vi "SP Convert SP TDMS Graphics to Display Cluster.vi"(8 "error in (no error)":errorcluster, 9 "S Parameter Formatting":T9 {"Plots"."Ch 2"."Reference" format="%#.2g"; "Plots"."Ch 2"."Display Data" items=["Data", "Memory", "Data/Memory"]; "Plots"."Ch 2"."Format" items=["Log Mag", "Phase", "Expanded Phase", "Delay", "Smith", "Polar", "Lin Mag", "SWR", "Loss", "Real", "Imaginary"]; "Plots"."Ch 2"."Scale" min=0.001 step=1.0 format="%#.2g"; "Plots"."Ch 2"."Position" min=0.0 max=10.0; "Plots"."Ch 1"."Reference" format="%#.2g"; "Plots"."Ch 1"."Display Data" items=["Data", "Memory", "Data/Memory"]; "Plots"."Ch 1"."Format" items=["Log Mag", "Phase", "Expanded Phase", "Delay", "Smith", "Polar", "Lin Mag", "SWR", "Loss", "Real", "Imaginary"]; "Plots"."Ch 1"."Scale" min=0.001 step=1.0 format="%#.2g"; "Plots"."Ch 1"."Position" min=0.0 max=10.0}) -> (0 "error out":errorcluster, 3 "Display":T1={"Lock Control"=FALSE, "Retain Settings"=TRUE, "Formatted Data"=FALSE, "Plot Orientation"=enum."Single", "Plot Controls"=[{"Trace Orientation"=enum."Overlay", "Frequency"={"Change Frequency"=FALSE, "Start"=500.0, "Stop"=1500.0, "Units"=enum."MHz"}, "Markers"=[], "Traces"=[]}, {"Trace Orientation"=enum."Overlay", "Frequency"={"Change Frequency"=FALSE, "Start"=500.0, "Stop"=1500.0, "Units"=enum."MHz"}, "Markers"=[], "Traces"=[]}, {"Trace Orientation"=enum."Overlay", "Frequency"={"Change Frequency"=FALSE, "Start"=500.0, "Stop"=1500.0, "Units"=enum."MHz"}, "Markers"=[], "Traces"=[]}, {"Trace Orientation"=enum."Overlay", "Frequency"={"Change Frequency"=FALSE, "Start"=500.0, "Stop"=1500.0, "Units"=enum."MHz"}, "Markers"=[], "Traces"=[]}]} {"Plot Controls"."Traces"."Reference" format="%#.2g"; "Plot Controls"."Traces"."Display Data" items=["Data", "Memory", "Data/Memory"]; "Plot Controls"."Traces"."Format" items=["Log Mag", "Phase", "Expanded Phase", "Delay", "Smith", "Polar", "Lin Mag", "SWR", "Loss", "Real", "Imaginary"]; "Plot Controls"."Traces"."Scale" min=0.001 step=1.0 format="%#.2g"; "Plot Controls"."Traces"."Position" min=0.0 max=10.0; "Plot Controls"."Frequency"."Stop" format="%.3g"; "Plot Controls"."Frequency"."Start" format="%.3g"})   [LabVIEW 2011]
uses:
  TypeDefs/SP Formatting.ctl
  TypeDefs/SP Plot Orientation.ctl
  TypeDefs/SP Plot.ctl
  TypeDefs/SP Trace Orientation.ctl
  TypeDefs/SP Display Trace Controls.ctl
  TypeDefs/SP Display Format.ctl
  TypeDefs/SP Display Data.ctl
  TypeDefs/SP Frequency Units.ctl
  TypeDefs/SP Display Parameters.ctl
  TypeDefs/SP Display Plot Controls Cluster.ctl
  TypeDefs/SP Marker Cluster.ctl
  TypeDefs/SP Marker Type.ctl
panel:
  # "Div"
  # "Div"
  # "Div"
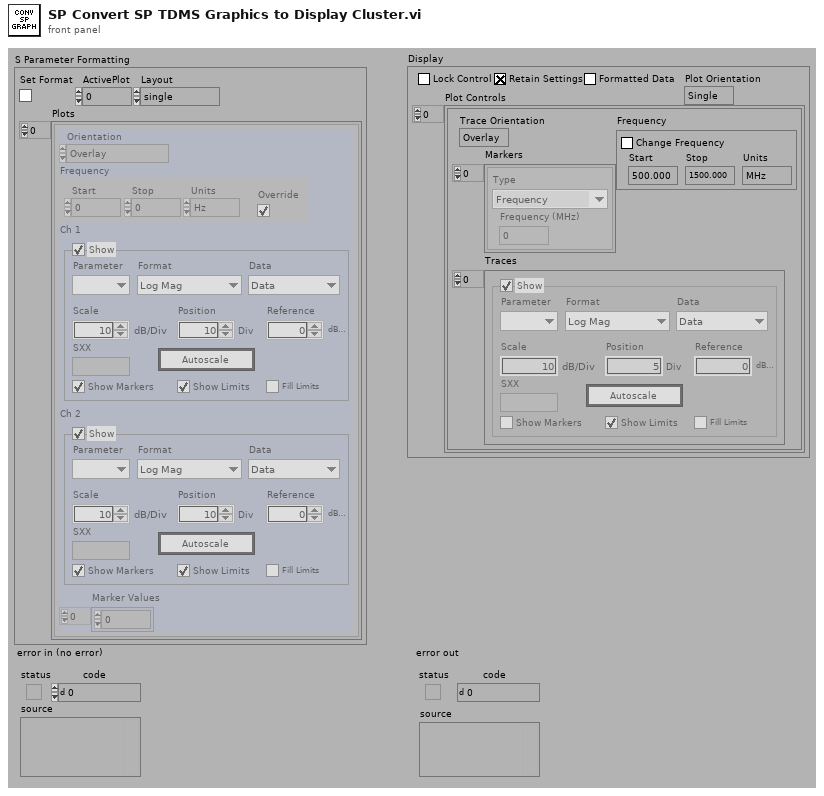
[diagram p1: front panel]
types:
  T1 = typedef "SP Display Parameters.ctl" = cluster{"Lock Control":bool, "Retain Settings":bool, "Formatted Data":bool, "Plot Orientation":enum32{"Single", "Dual", "Quad"}, "Plot Controls":T2[]}
  T2 = typedef "SP Display Plot Controls Cluster.ctl" = cluster{"Trace Orientation":enum32{"Overlay", "Split"}, "Frequency":cluster{"Change Frequency":bool, "Start":dbl, "Stop":dbl, "Units":T3}, "Markers":T4[], "Traces":T6[]}
  T3 = typedef "SP Frequency Units.ctl" = enum16{"Hz", "kHz", "MHz", "GHz", "Points"}
  T4 = typedef "SP Marker Cluster.ctl" = cluster{"Type":T5, "Frequency (MHz)":dbl}
  T5 = typedef "SP Marker Type.ctl" = enum16{"Frequency", "Trace Maximum", "Trace Minimum", "Limit Maximum", "Limit Minimum"}
  T6 = typedef "SP Display Trace Controls.ctl" = cluster{"Trace On":bool, "Measure":i32, "Format":T7, "Autoscale":bool, "Reference":dbl, "\nRefUnit":string, "Position":dbl, "Scale":dbl, "ScaleUnit":string, "LimitOn":bool, "LimitFill":bool, "Display Data":T8, "Show Markers":bool, "SXX":string}
  T7 = typedef "SP Display Format.ctl" = i32
  T8 = typedef "SP Display Data.ctl" = u16
  T9 = typedef "SP Formatting.ctl" = cluster{"Set Format":bool, "Layout":T10, "ActivePlot":i32, "Plots":T11[]}
  T10 = typedef "SP Plot Orientation.ctl" = enum32{"single", "dual", "quad"}
  T11 = typedef "SP Plot.ctl" = cluster{"Orientation":T12, "Ch 1":T6, "Ch 2":T6, "Frequency":cluster{"Start":dbl, "Stop":dbl, "Units":T3, "Override":bool}, "Marker Values":dbl[]}
  T12 = typedef "SP Trace Orientation.ctl" = enum32{"Overlay", "Split"}
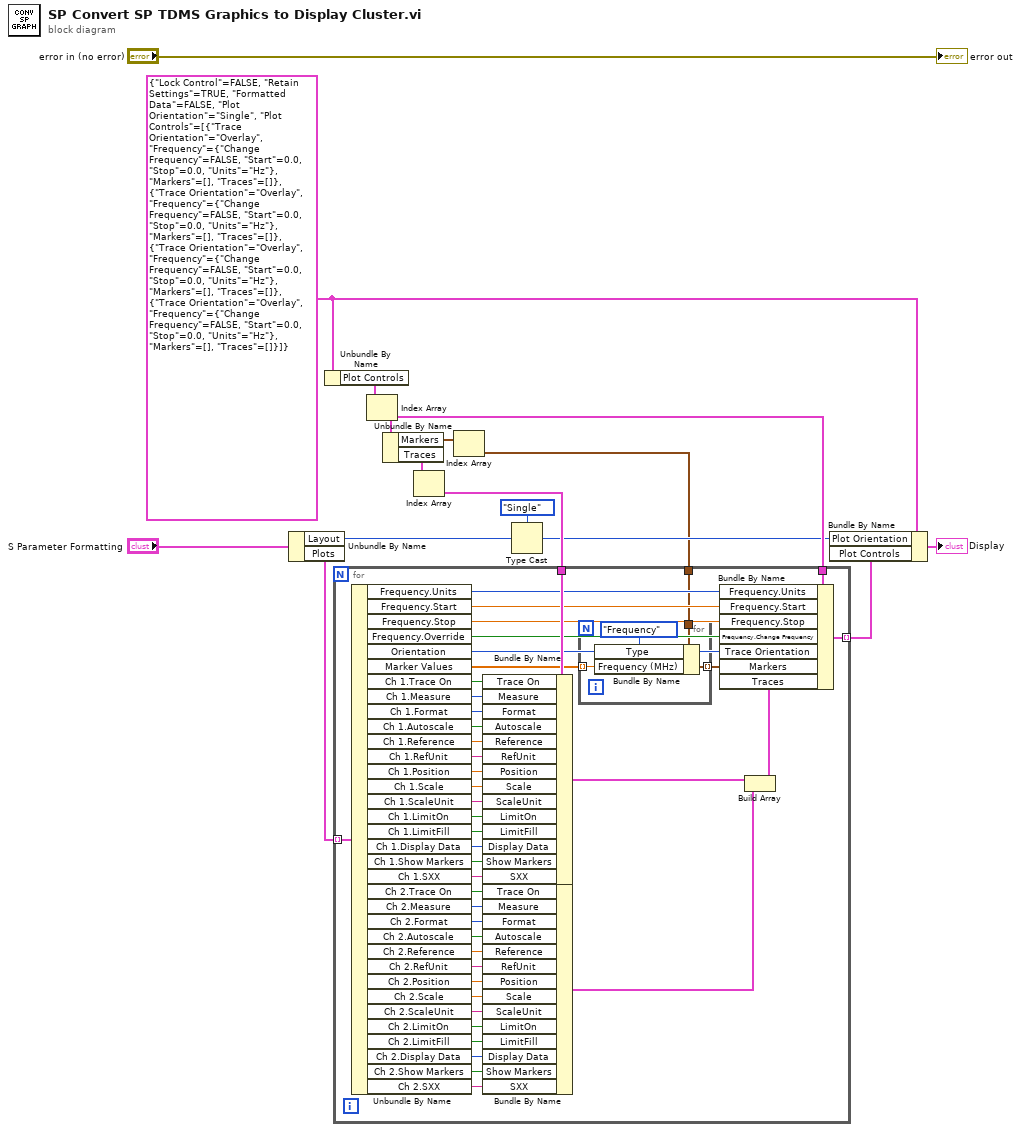
[diagram p0: block diagram]
diagram:
  w8 = T1 {"Lock Control"=FALSE, "Retain Settings"=TRUE, "Formatted Data"=FALSE, "Plot Orientation"=enum."Single", "Plot Controls"=[{"Trace Orientation"=enum."Overlay", "Frequency"={"Change Frequency"=FALSE, "Start"=0.0, "Stop"=0.0, "Units"=enum."Hz"}, "Markers"=[], "Traces"=[]}, {"Trace Orientation"=enum."Overlay", "Frequency"={"Change Frequency"=FALSE, "Start"=0.0, "Stop"=0.0, "Units"=enum."Hz"}, "Markers"=[], "Traces"=[]}, {"Trace Orientation"=enum."Overlay", "Frequency"={"Change Frequency"=FALSE, "Start"=0.0, "Stop"=0.0, "Units"=enum."Hz"}, "Markers"=[], "Traces"=[]}, {"Trace Orientation"=enum."Overlay", "Frequency"={"Change Frequency"=FALSE, "Start"=0.0, "Stop"=0.0, "Units"=enum."Hz"}, "Markers"=[], "Traces"=[]}]} ("Display")
  n1 = Unbundle By Name("S Parameter Formatting") -> ("Layout"=w6:T10, "Plots"=w13:T11[])
  n2 = Unbundle By Name(w8) -> ("Plot Controls"=w12:T2[])
  n3 = Index Array(array=w12) -> (element=w9:T2)  [unwired: 1 in]
  n4 = Unbundle By Name(w9) -> ("Markers"=w2:T4[], "Traces"=w11:T6[])
  n5 = Index Array(array=w11) -> (element=w10:T6)  [unwired: 1 in]
  n6 = Index Array(array=w2) -> (element=w1:T4)  [unwired: 1 in]
  n7 = for {
    tunnel: w13 -> [w58] mode=indexing
    tunnel: w10 -> [w29]
    tunnel: w9 -> [w28]
    tunnel: [w20] -> w7 mode=indexing
    tunnel: w1 -> [w17]
    n8 = Unbundle By Name(w58) -> ("Frequency.Units"=w27:T3, "Frequency.Start"=w26:dbl, "Frequency.Stop"=w25:dbl, "Frequency.Override"=w19:bool, "Orientation"=w24:T12, "Marker Values"=w18:dbl[], "Ch 1.Trace On"=w57:bool, "Ch 1.Measure"=w56:i32, "Ch 1.Format"=w55:T7, "Ch 1.Autoscale"=w54:bool, "Ch 1.Reference"=w53:dbl, "Ch 1.RefUnit"=w52:string, "Ch 1.Position"=w51:dbl, "Ch 1.Scale"=w50:dbl, "Ch 1.ScaleUnit"=w49:string, "Ch 1.LimitOn"=w48:bool, "Ch 1.LimitFill"=w47:bool, "Ch 1.Display Data"=w46:T8, "Ch 1.Show Markers"=w45:bool, "Ch 1.SXX"=w44:string, "Ch 2.Trace On"=w43:bool, "Ch 2.Measure"=w42:i32, "Ch 2.Format"=w41:T7, "Ch 2.Autoscale"=w40:bool, "Ch 2.Reference"=w39:dbl, "Ch 2.RefUnit"=w38:string, "Ch 2.Position"=w37:dbl, "Ch 2.Scale"=w36:dbl, "Ch 2.ScaleUnit"=w35:string, "Ch 2.LimitOn"=w34:bool, "Ch 2.LimitFill"=w33:bool, "Ch 2.Display Data"=w32:T8, "Ch 2.Show Markers"=w31:bool, "Ch 2.SXX"=w30:string)
    n9 = Bundle By Name(cluster=w29, "Trace On"=w57, "Measure"=w56, "Format"=w55, "Autoscale"=w54, "Reference"=w53, "RefUnit"=w52, "Position"=w51, "Scale"=w50, "ScaleUnit"=w49, "LimitOn"=w48, "LimitFill"=w47, "Display Data"=w46, "Show Markers"=w45, "SXX"=w44) -> (w23:T6)
    n10 = Bundle By Name(cluster=w29, "Trace On"=w43, "Measure"=w42, "Format"=w41, "Autoscale"=w40, "Reference"=w39, "RefUnit"=w38, "Position"=w37, "Scale"=w36, "ScaleUnit"=w35, "LimitOn"=w34, "LimitFill"=w33, "Display Data"=w32, "Show Markers"=w31, "SXX"=w30) -> (w21:T6)
    n11 = for {
      tunnel: w18 -> [w61] mode=indexing
      tunnel: w17 -> [w62]
      tunnel: [w59] -> w16 mode=indexing
      n12 = Bundle By Name(cluster=w62, "Type"=SP_Marker_Type."Frequency", "Frequency (MHz)"=w61) -> (w59:T4)
    }
    n13 = Build Array(w23, w21) -> (w22:T6[])
    n14 = Bundle By Name(cluster=w28, "Frequency.Units"=w27, "Frequency.Start"=w26, "Frequency.Stop"=w25, "Frequency.Change Frequency"=w19, "Trace Orientation"=w24, "Markers"=w16, "Traces"=w22) -> (w20:T2)
  }
  n15 = Type Cast(type=enum32{"Single", "Dual", "Quad"}."Single" ("Plot Orientation"), x=w6) -> (*(type *) &x=w5:enum32{"Single", "Dual", "Quad"})
  n16 = Bundle By Name(cluster=w8, "Plot Orientation"=w5, "Plot Controls"=w7) -> (→"Display":T1)
  "error out" <- "error in (no error)"
